vi "Write Channel to TDMS Log File (Waveform).vi"(6 "Waveform Data":waveform(dbl), 8 "error in (no error)":errorcluster, 9 "Channel Name in":string, 10 "Group Name in":string, 11 "TDMS Log File in":refnum<class "TDMS Log File.lvclass">) -> (0 "error out":errorcluster, 3 "TDMS Log File out":refnum<class "TDMS Log File.lvclass">)   [LabVIEW 2015, in "TDMS Log File.lvclass"]
uses:
  TDMS Log File.lvclass
  TDMS Log File.lvclass/TDMS Log File.ctl
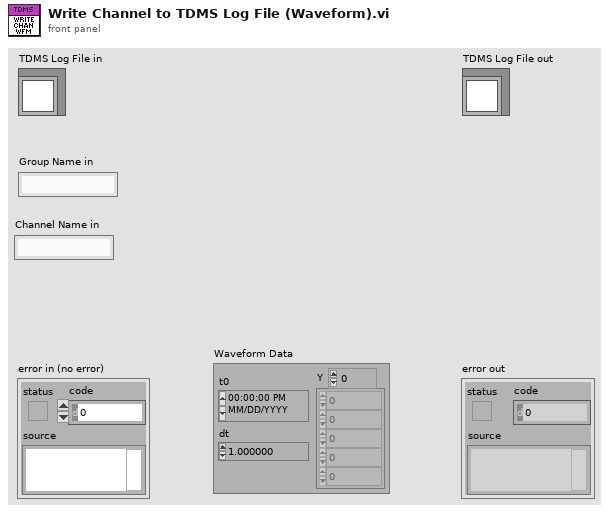
[diagram p1: front panel]
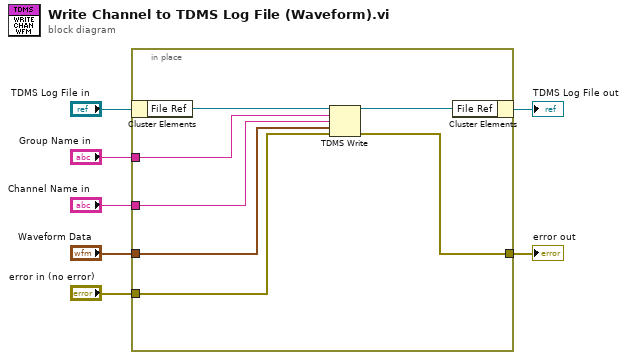
[diagram p0: block diagram]
diagram:
  n1 = in-place {
    in-place-border: "Group Name in" -> [w13]
    in-place-border: "Channel Name in" -> [w12]
    in-place-border: "Waveform Data" -> [w11]
    in-place-border: "error in (no error)" -> [w9]
    in-place-border: [w8] -> w4
    n2 = in-place-cluster #1("TDMS Log File in") -> ("File Ref"=w14:refnum<k34>)
    n3 = TDMS Write(0:w14, 5:w13, 7:w12, 9:w11, 11:w9) -> (4:w10:refnum<k34>, 15:w8:errorcluster)  [unwired: 1 in, 2 out]
    n4 = in-place-cluster #1("File Ref"=w10) -> (→"TDMS Log File out":refnum<class "TDMS Log File.lvclass">)
  }
  "error out" <- w4
